vi "laserControl.vi"() -> ()   [LabVIEW 2017]
uses:
  <vilib>/DAQmx/write.llb/DAQmx Write (Digital 1D U8 1Chan NSamp).vi
  <vilib>/DAQmx/create/channels.llb/DAQmx Create Channel (DO-Digital Output).vi
  <vilib>/DAQmx/configure/timing.llb/DAQmx Timing (Sample Clock).vi
  <vilib>/DAQmx/miscellaneous.llb/DAQmx Fill In Error Info.vi
panel:
  in  "stop":bool
  out "Array 2":i32[](array[numeric])
  out "element":u8
  out "Array":u8[](array[numeric])
  in  "rep rate division":u16=2
  in  "pulses":u16=10
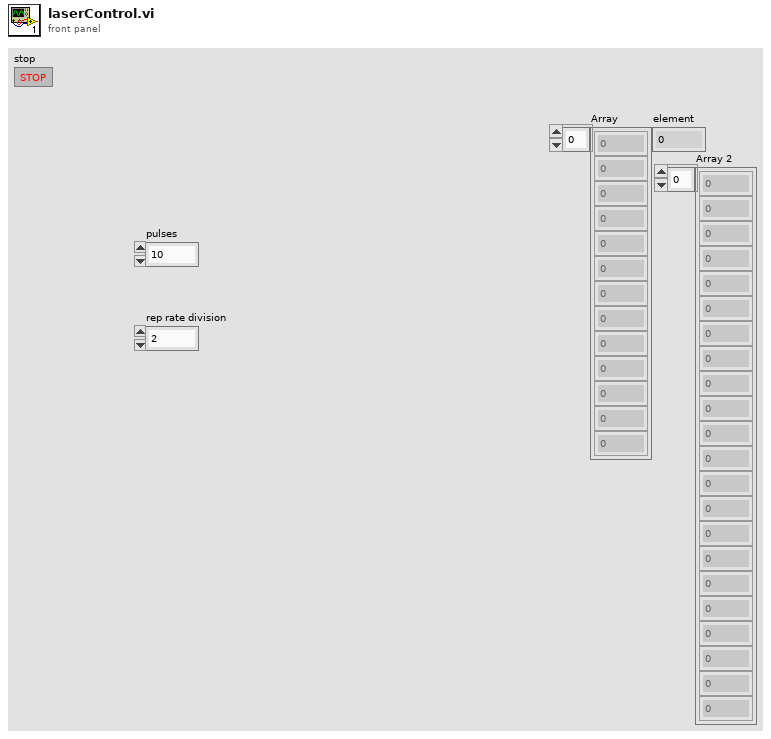
[diagram p1: front panel]
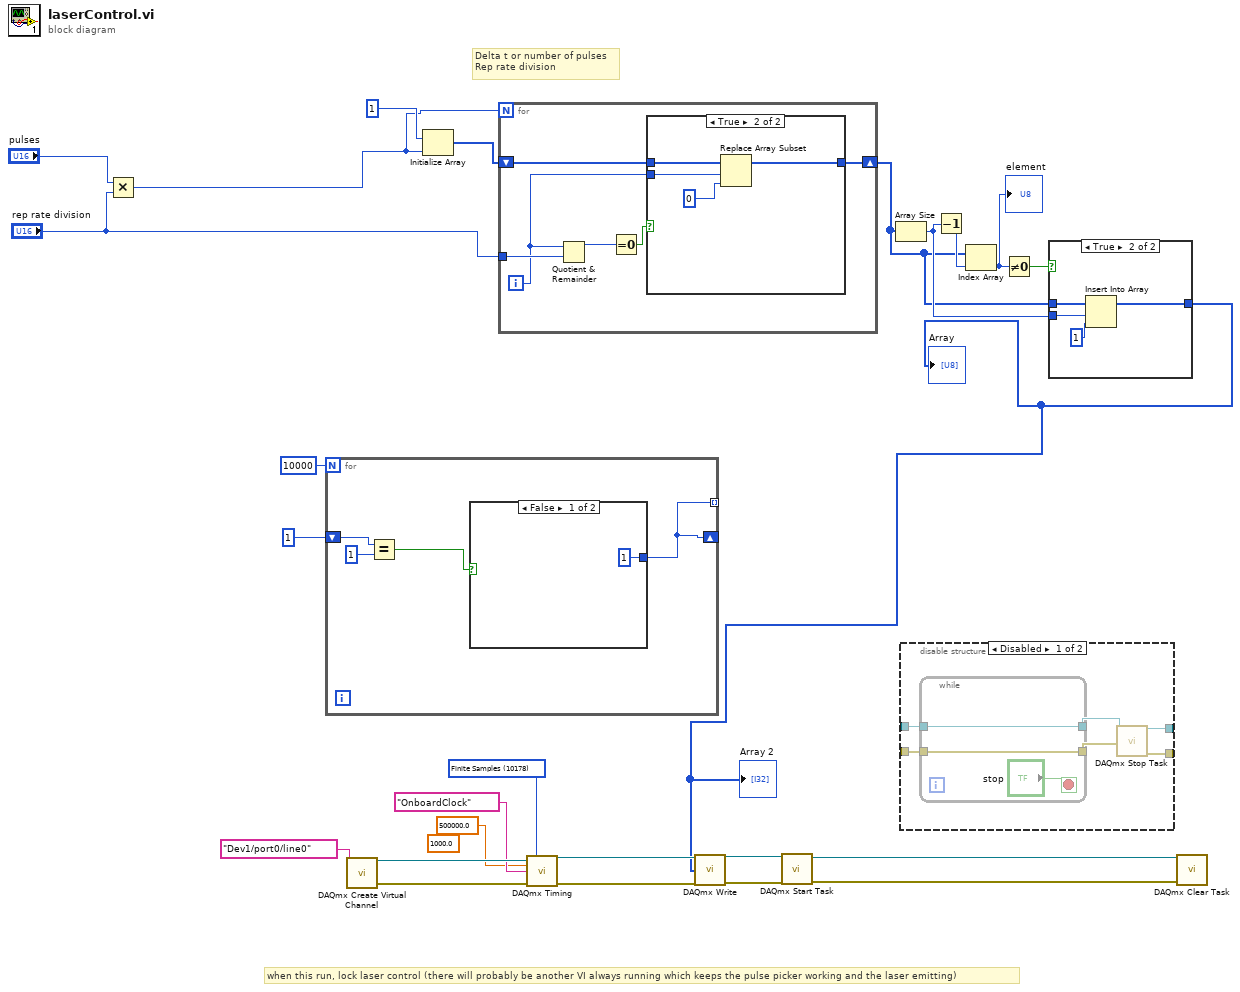
[diagram p0: block diagram]
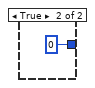
[diagram p3: hidden frame]
diagram:
  (unwired) 1000.0 ("rate")
  w13 = 10178 items=["Finite Samples"=10178, "Continuous Samples"=10123, "Hardware Timed Single Point"=12522] ("sample mode")
  # "when this run, lock laser control (there will probably be another VI always running which keeps the pulse picker working and the laser emitting)"
  # "Delta t or number of pulses\nRep rate division"
  n1 = Multiply(x="pulses", y="rep rate division") -> (x*y=w21:u16)
  n2 = for {
    N: 10000 -> [_]
    shift-right: [w26] -> _
    shift-left: 1 -> [w29]
    tunnel: [w26] -> _ mode=indexing
    n3 = Equal?(x=w29, y=1) -> (x = y?=w27:bool)
    n4 = case shown="False" w27 {
      tunnel: [1 0] -> w26
      frame False {
      }
      frame True {
      }
    }
  }
  n5 = call-poly <vilib>:"DAQmx Create Virtual Channel.vi"("lines"=tag "Dev1/port0/line0") -> ("task out"=w15:refnum<k21>, "error out"=w8:errorcluster)  [unwired: 13 in]
  n6 = Initialize Array(u8 1, w21) -> (w25:u8[])
  n7 = for {
    N: w21 -> [_]
    tunnel: "rep rate division" -> [w37]
    shift-right: [w33] -> w4
    shift-left: w25 -> [w35]
    i -> [w34]
    n8 = Quotient & Remainder(x=w34, y=w37) -> (x-y*floor(x/y)=w36:i32)  [unwired: 1 out]
    n9 = Equal To 0?(x=w36) -> (x = 0?=w32:bool)
    n10 = case shown="True" w32 {
      tunnel: w35 -> [w38 w42]
      tunnel: w34 -> [_ w41]
      tunnel: [w38 w39] -> w33
      frame False {
      }
      frame True {
        n11 = Replace Array Subset(array=w42, new element=u8 0, index=w41) -> (w39:u8[])
      }
    }
  }
  n12 = call-poly <vilib>:"DAQmx Timing.vi"("task/channels in"=w15, "sample mode"=w13, "rate"=500000.0, "source"=tag "OnboardClock", "error in"=w8) -> ("task out"=w12:refnum<k21>, "error out"=w9:errorcluster)  [unwired: 9 in]
  n13 = Array Size(array=w4) -> (size(s)=w18:i32)
  n14 = disable-structure shown="Disabled" {
    disable-tunnel: _ -> [w48 _]
    disable-tunnel: [w46 _] -> _
    disable-tunnel: _ -> [w45 _]
    disable-tunnel: [w43 _] -> _
    frame Disabled {
      n15 = while {
        tunnel: w48 -> [w50]
        tunnel: [w50] -> w47
        tunnel: w45 -> [w49]
        tunnel: [w49] -> w44
        stop <- "stop" stop-if-true
      }
      n16 = call <vilib>:"DAQmx Stop Task.vi"("task/channels in"=w47, "error in"=w44) -> ("task out"=w46:refnum<k21>, "error out"=w43:errorcluster)  [unwired: 12 in]
    }
    frame Enabled {
    }
  }
  n17 = Decrement(x=w18) -> (x-1=w17:i32)
  n18 = Index Array(array=w4, index=w17) -> (element=w20:u8)
  "element" <- w20
  n19 = Not Equal To 0?(x=w20) -> (x != 0?=w19:bool)
  n20 = case shown="True" w19 {
    tunnel: w4 -> [w52 w56]
    tunnel: w18 -> [_ w55]
    tunnel: [w52 w53] -> w1
    frame False {
    }
    frame True {
      n21 = Insert Into Array(array=w56, index=w55, new element=u8 1 ("new element/subarray")) -> (w53:u8[])
    }
  }
  "Array" <- w1
  "Array 2" <- w1
  n22 = call-poly <vilib>:"DAQmx Write.vi"("task/channels in"=w12, "data"=w1, "error in"=w9) -> ("task out"=w11:refnum<k21>, "error out"=w10:errorcluster)  [unwired: 10 in, 1 out]
  n23 = call <vilib>:"DAQmx Start Task.vi"("task/channels in"=w11, "error in"=w10) -> ("task out"=w3:refnum<k21>, "error out"=w2:errorcluster)  [unwired: 12 in]
  n24 = call <vilib>:"DAQmx Clear Task.vi"("task in"=w3, "error in"=w2) -> ()  [unwired: 13 in, 1 out]
